vi "testing parameters.vi"() -> ()   [LabVIEW 2017]
uses:
  b0ea6400-f917-4b5c-8b78-857e45cd8847.vi
  <vilib>/addons/database/Connection.llb/DB Tools Open Connec (Path).vi
  <vilib>/addons/database/NI_Database_API.lvlib
panel:
  out "index of element":i32
  out "output array":string[](array[string])
  out "resulting string":string
  in  "condition":string[](array[string])
  in  "data 2":string[][](array[string])
  out "data":string[][](array[string])
  out "error out 4":errorcluster
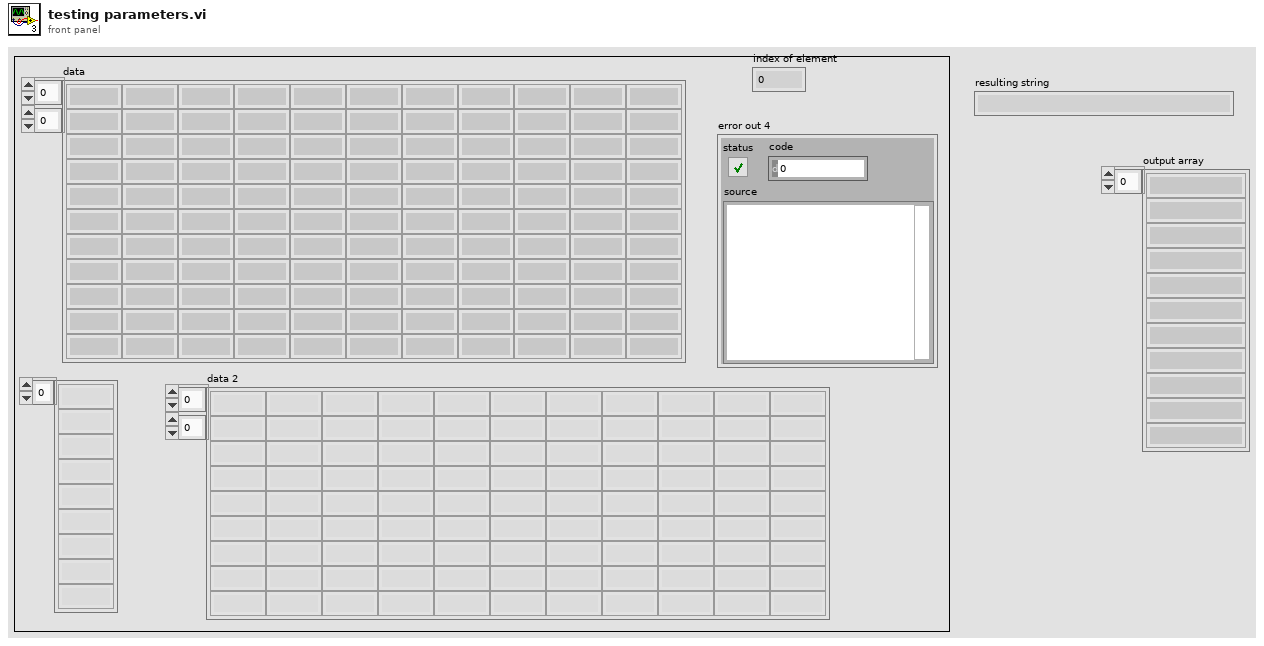
[diagram p1: front panel]
types:
  T1 = typedef "NI_Database_API.lvlib/Conn ObjectReference.ctl" = refnum<k1>
  T2 = cluster{"[0]":string, "[1]":string, "[2]":string, "[3]":string, "[4]":string, "[5]":string, "[6]":string, "[7]":string}
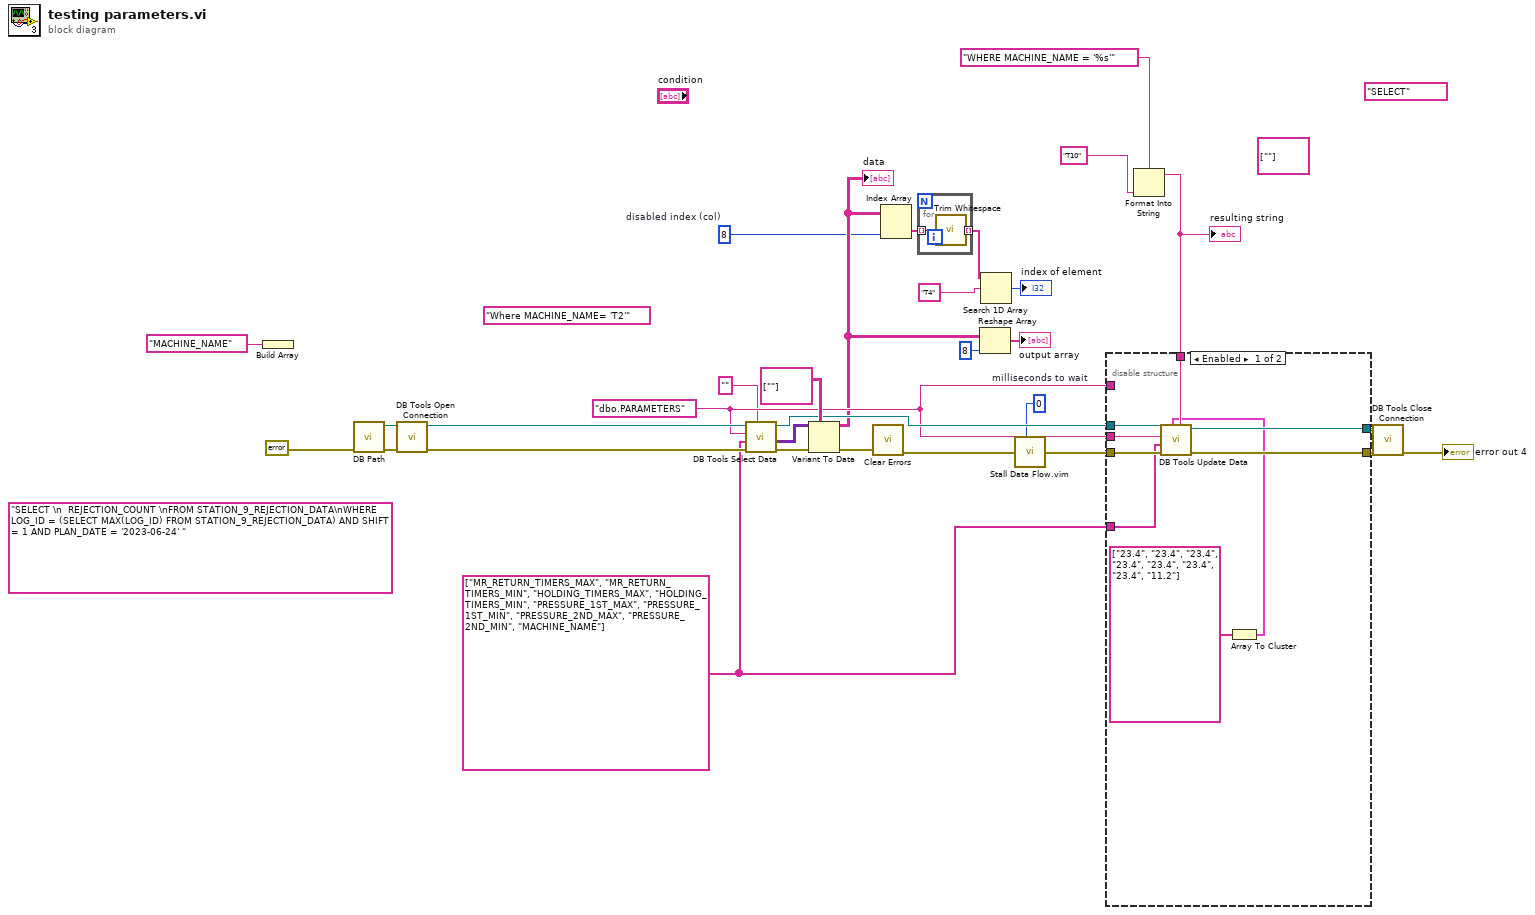
[diagram p0: block diagram]
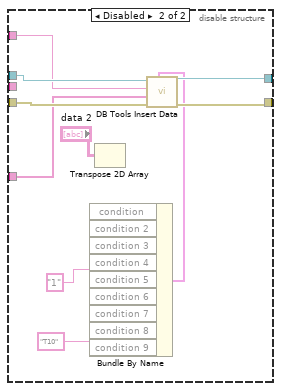
[diagram p2: hidden frame]
diagram:
  w6 = 8  # disabled index (col)
  (unwired) string[][] [[""]]
  w13 = u32 0  # milliseconds to wait
  w10 = string[] ["MR_RETURN_TIMERS_MAX", "MR_RETURN_TIMERS_MIN", "HOLDING_TIMERS_MAX", "HOLDING_TIMERS_MIN", "PRESSURE_1ST_MAX", "PRESSURE_1ST_MIN", "PRESSURE_2ND_MAX", "PRESSURE_2ND_MIN", "MACHINE_NAME"] ("String")
  (unwired) "Where MACHINE_NAME= 'T2'" ("condition")
  (unwired) "SELECT"
  (unwired) "SELECT \n  REJECTION_COUNT \nFROM STATION_9_REJECTION_DATA\nWHERE LOG_ID = (SELECT MAX(LOG_ID) FROM STATION_9_REJECTION_DATA) AND SHIFT = 1 AND PLAN_DATE = '2023-06-24' " ("SQL query")
  w12 = "dbo.PARAMETERS" ("table")
  n1 = Build Array("MACHINE_NAME" ("String")) -> ()  [unwired: 1 out]
  n2 = call "DB Path.vi"("error in"=errorcluster {"status"=FALSE, "code"=0, "source"=""} ("error in (no error)")) -> ("error out"=w26:errorcluster, "DB Path"=w27:path)  [unwired: 9 in]
  n3 = call-poly <vilib>:"DB Tools Open Connection.vi"("error in (no error)"=w26, "connection information"=w27) -> ("error out"=w19:errorcluster, "connection reference"=w25:T1)  [unwired: 6 in]
  n4 = call <vilib>:"DB Tools Select Data.vi"("condition"="", "error in (no error)"=w19, "columns"=w10, "table"=w12, "connection reference"=w25) -> ("error out"=w31:errorcluster, "data"=w30:variant[][], "connection reference out"=w22:T1)  [unwired: 1 in]
  n5 = Variant To Data(error in=w31, type=string[][] [[""]], Variant=w30) -> (data=w9:string[][], error out=w28:errorcluster)
  "data" <- w9
  n6 = call <vilib>:"Clear Errors.vi"("error in (no error)"=w28) -> ("error out"=w18:errorcluster)  [unwired: 5 in, 1 out]
  n7 = Index Array(array=w9, index (col)=w6) -> (element=w5:string[])  [unwired: 1 in]
  n8 = for {
    tunnel: w5 -> [w33] mode=indexing
    tunnel: [w32] -> w1 mode=indexing
    n9 = call <vilib>:"Trim Whitespace.vi"("string"=w33) -> ("trimmed string"=w32:string)  [unwired: 1 in]
  }
  n10 = Reshape Array(w9, 8 ("dimension size")) -> (→"output array":string[])
  n11 = Search 1D Array(1D array=w1, element="T4" ("condition")) -> (index of element=→"index of element":i32)  [unwired: 1 in]
  n12 = call "Stall Data Flow.vim"("value in"=w18, "milliseconds to wait"=w13) -> ("value out"=w14:errorcluster)  [unwired: 1 out]
  n13 = Format Into String(format string="WHERE MACHINE_NAME = '%s'" ("condition"), "T10" ("condition")) -> (resulting string=w16:string)  [unwired: 2 in, 1 out]
  "resulting string" <- w16
  n14 = disable-structure shown="Enabled" {
    disable-tunnel: [w42 w52] -> w23
    disable-tunnel: w22 -> [w41 w50]
    disable-tunnel: [w40 w51] -> w21
    disable-tunnel: w12 -> [w39 _]
    disable-tunnel: w16 -> [w38 _]
    disable-tunnel: w14 -> [w37 w53]
    disable-tunnel: w10 -> [w36 w49]
    disable-tunnel: w12 -> [_ w48]
    frame Enabled {
      n15 = Array To Cluster(array=string[] ["23.4", "23.4", "23.4", "23.4", "23.4", "23.4", "23.4", "11.2"]) -> (cluster=w34:T2)
      n16 = call <vilib>:"DB Tools Update Data.vi"("condition"=w38, "data"=w34, "error in (no error)"=w37, "columns"=w36, "table"=w39, "connection reference"=w41) -> ("error out"=w42:errorcluster, "connection reference out"=w40:T1)  [unwired: 4 in]
    }
    frame Disabled {
      w44 = "1" ("condition")
      n17 = Bundle By Name("condition"=w44, "condition 2"=w44, "condition 3"=w44, "condition 4"=w44, "condition 5"=w44, "condition 6"=w44, "condition 7"=w44, "condition 8"=w44, "condition 9"="T10" ("condition")) -> (w46:cluster{}, w43:cluster{})
      n18 = Transpose 2D Array(2D array="data 2") -> ()  [unwired: 1 out]
      n19 = call <vilib>:"DB Tools Insert Data.vi"("data"=w46, "error in (no error)"=w53, "columns"=w49, "table"=w48, "connection reference"=w50) -> ("error out"=w52:errorcluster, "connection reference out"=w51:T1)  [unwired: 5 in]
    }
  }
  n20 = call <vilib>:"DB Tools Close Connection.vi"("error in (no error)"=w23, "connection reference"=w21) -> ("error out"=→"error out 4":errorcluster)  [unwired: 5 in]
